vi "calibration_test_R.vi"(7 "i_pos_thres":i32, 8 "Reset zero":bool, 10 "Hip angle":dbl) -> (0 "zero position":dbl, 1 "diff":dbl, 2 "min":dbl, 3 "max":dbl)   [LabVIEW 2019]
uses:
  <vilib>/functionblocks/Edge Detection/One Shot Rising with Input/One Shot Rising with Input.vi
  <vilib>/functionblocks/FB Core/FB Core.xnode
  <vilib>/functionblocks/NI_FunctionBlock Libraries.lvlib
panel:
  out "i_pos":i32
  out "min_temp":dbl
  out "decreasing counter":i32
  out "increasing counter":i32
  out "max_temp":dbl
  out "hip angle < zero":bool
  out "iteraction":i32
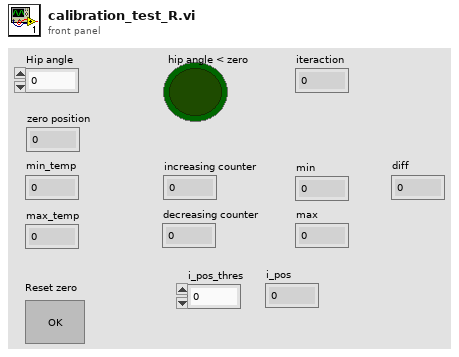
[diagram p1: front panel]
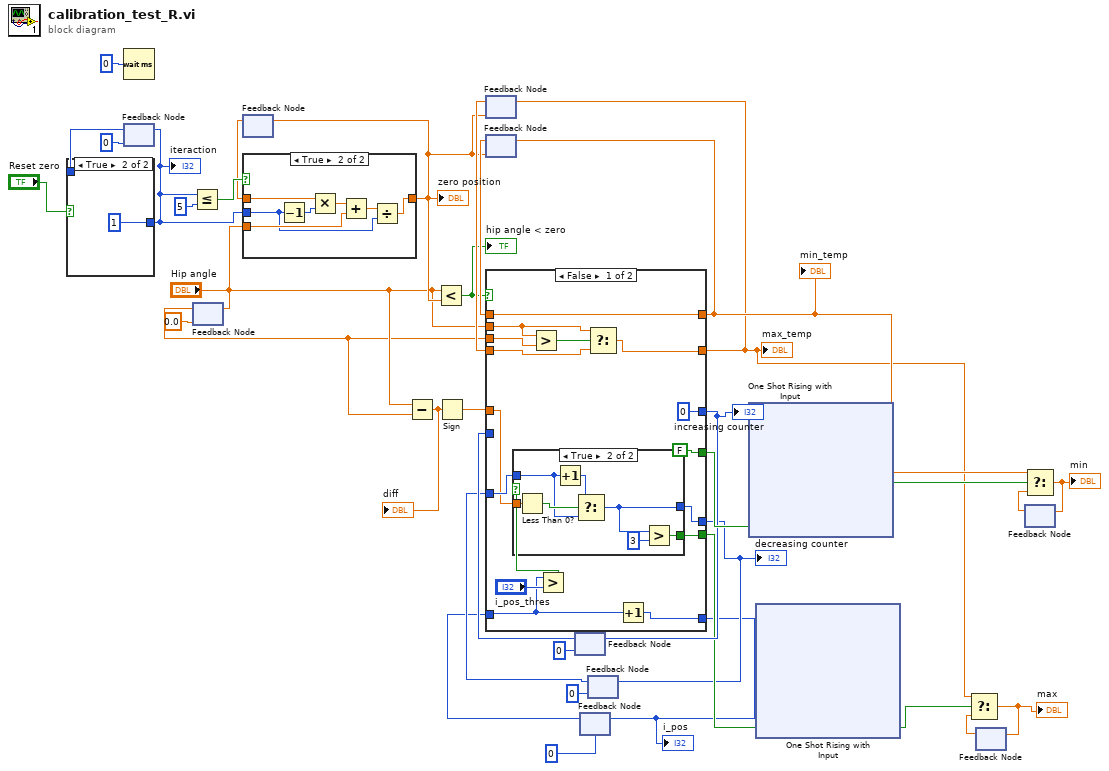
[diagram p0: block diagram]
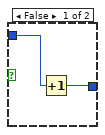
[diagram p2: hidden frame]
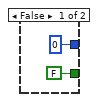
[diagram p3: hidden frame]
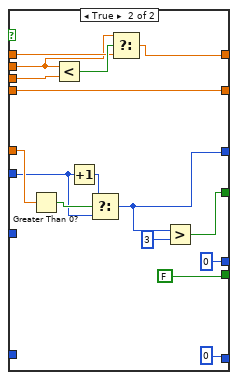
[diagram p4: hidden frame]
diagram:
  n1 = Wait (ms)(milliseconds to wait=u32 0) -> ()  [unwired: 1 out]
  n2 = feedback #1(0) -> (w30:i32)
  n3 = case shown="True" "Reset zero" {
    tunnel: [w38 1] -> w31
    tunnel: w30 -> [w37 _]
    frame False {
      n4 = Increment(x=w37) -> (x+1=w38:i32)
    }
    frame True {
    }
  }
  "iteraction" <- w31
  n5 = feedback-in #1(w31) -> ()
  n6 = Less Or Equal?(x=w31, y=5) -> (x <= y?=w34:bool)
  n7 = feedback #2(0.0 ("Scalar")) -> (w23:dbl)
  n8 = feedback-in #2("Hip angle") -> ()
  n9 = feedback #3() -> (w33:dbl)  [unwired: 1 in]
  n10 = case shown="True" w34 {
    tunnel: "Hip angle" -> [_ w45]
    tunnel: [w40 w47] -> w27
    tunnel: w33 -> [w40 w44]
    tunnel: w31 -> [_ w43]
    frame False {
    }
    frame True {
      n11 = Decrement(x=w43) -> (x-1=w42:i32)
      n12 = Multiply(x=w44, y=w42) -> (x*y=w41:dbl)
      n13 = Add(x=w41, y=w45) -> (x+y=w46:dbl)
      n14 = Divide(x=w46, y=w43) -> (x/y=w47:dbl)
    }
  }
  "zero position" <- w27
  n15 = feedback-in #3(w27) -> ()
  n16 = Subtract(x="Hip angle", y=w23) -> (x-y=w4:dbl)
  "diff" <- w4
  n17 = Less?(x="Hip angle", y=w27) -> (x < y?=w26:bool)
  "hip angle < zero" <- w26
  n18 = Sign(1:w4) -> (0:w22:dbl)
  n19 = feedback #4(w27) -> (w28:dbl)
  n20 = feedback #5(w27) -> (w29:dbl)
  n21 = feedback #6(0) -> (w15:i32)
  n22 = feedback #7(0) -> (w2:i32)
  n23 = feedback #8(0) -> (w6:i32)
  n24 = case shown="False" w26 {
    tunnel: "Hip angle" -> [w60 w85]
    tunnel: [w58 w87] -> w21
    tunnel: w29 -> [w58 w86]
    tunnel: [w62 w83] -> w5
    tunnel: w28 -> [w61 w83]
    tunnel: w23 -> [w59 w84]
    tunnel: w22 -> [w53 w82]
    tunnel: [FALSE w74] -> w17
    tunnel: [0 w78] -> w16
    tunnel: w15 -> [_ w77]
    tunnel: [w48 FALSE] -> w12
    tunnel: [w55 0] -> w8
    tunnel: w6 -> [w54 _]
    tunnel: [w52 0] -> w1
    tunnel: w2 -> [w50 _]
    frame False {
      n25 = Greater?(x=w60, y=w59) -> (0:w63:bool)
      n26 = Greater?(x=w50, y="i_pos_thres") -> (0:w49:bool)
      n27 = case shown="True" w49 {
        tunnel: [0 w69] -> w55
        tunnel: w54 -> [_ w68]
        tunnel: w53 -> [_ w67]
        tunnel: [FALSE w66] -> w48
        frame False {
        }
        frame True {
          n28 = Less Than 0?(x=w67) -> (x < 0?=w72:bool)
          n29 = Increment(x=w68) -> (x+1=w71:i32)
          n30 = Select(t=w71, s=w72, f=w68) -> (s? t:f=w69:i32)
          n31 = Greater?(x=w69, y=3) -> (0:w66:bool)
        }
      }
      n32 = Select(t=w60, s=w63, f=w61) -> (s? t:f=w62:dbl)
      n33 = Increment(x=w50) -> (x+1=w52:i32)
    }
    frame True {
      n34 = Greater Than 0?(x=w82) -> (x > 0?=w81:bool)
      n35 = Less?(x=w85, y=w84) -> (x < y?=w88:bool)
      n36 = Increment(x=w77) -> (x+1=w80:i32)
      n37 = Select(t=w80, s=w81, f=w77) -> (s? t:f=w78:i32)
      n38 = Select(t=w85, s=w88, f=w86) -> (s? t:f=w87:dbl)
      n39 = Greater?(x=w78, y=3) -> (0:w74:bool)
    }
  }
  "max_temp" <- w5
  "increasing counter" <- w16
  "decreasing counter" <- w8
  "min_temp" <- w21
  "i_pos" <- w1
  n40 = feedback-in #4(w5) -> ()
  n41 = feedback-in #5(w21) -> ()
  n42 = feedback-in #6(w16) -> ()
  n43 = feedback-in #7(w1) -> ()
  n44 = feedback-in #8(w8) -> ()
  n45 = xnode "One Shot Rising with Input"("input"=w17) -> ("output"=w18:bool)  [unwired: 1 in, 1 out]
  n46 = xnode "One Shot Rising with Input"("input"=w12) -> ("output"=w11:bool)  [unwired: 1 in, 1 out]
  n47 = feedback #9() -> (w9:dbl)  [unwired: 1 in]
  n48 = Select(t=w5, s=w11, f=w9) -> (s? t:f=w10:dbl)
  "max" <- w10
  n49 = feedback-in #9(w10) -> ()
  n50 = feedback #10() -> (w19:dbl)  [unwired: 1 in]
  n51 = Select(t=w21, s=w18, f=w19) -> (s? t:f=w20:dbl)
  "min" <- w20
  n52 = feedback-in #10(w20) -> ()
